vi "key_jiaoyan.vi"(10 "key_client":string, 11 "gonghao":string) -> (0 "jy":bool, 2 "error":errorcluster caption="错误输出")   [LabVIEW 2017, in "Lib_code.lvlib"]
uses:
  Lib_code.lvlib
panel:
  in  "簇":cluster{"key":string, "time":i64}
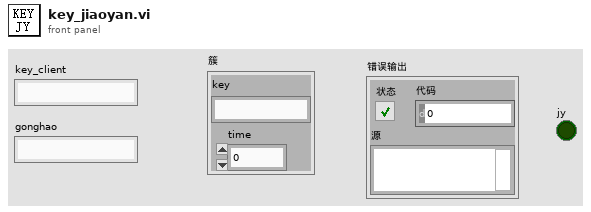
[diagram p1: front panel]
types:
  T1 = enum16{"big-endian, network order", "native, host order", "little-endian"}
  T2 = enum16{"open", "replace", "create", "open or create", "replace or create", "replace or create with confirmation"}
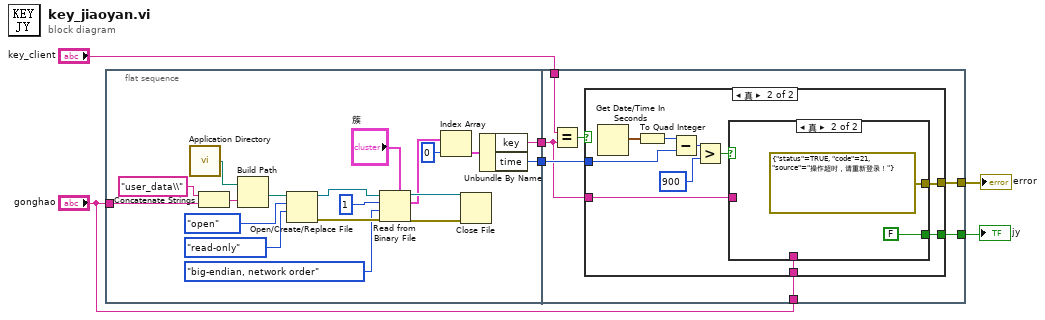
[diagram p0: block diagram]
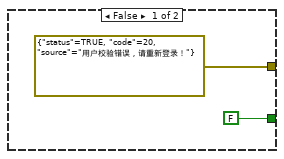
[diagram p2: hidden frame]
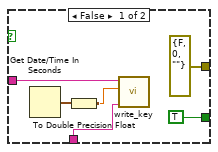
[diagram p3: hidden frame]
diagram:
  n1 = flat-sequence {
    tunnel: "gonghao" -> [w11]
    tunnel: [w10] -> w6
    tunnel: [w9] -> w3
    tunnel: w6 -> [w27]
    tunnel: "key_client" -> [w32]
    tunnel: [w30] -> w4
    tunnel: w3 -> [w29]
    tunnel: [w28] -> w2
    tunnel: "gonghao" -> [w26]
    frame #0 {
      n2 = call <vilib>:"Application Directory.vi"() -> ("Application Directory"=w25:path)
      n3 = Concatenate Strings("user_data\\" ("字符串"), w11) -> (w24:string)
      n4 = Build Path(base path=w25, name or relative path=w24) -> (appended path=w22:path)
      n5 = Open/Create/Replace File(file path (use dialog)=w22, operation (0:open)=T2."open" ("操作(0:open)"), access (0:read/write)=enum16{"read/write", "read-only", "write-only"}."read-only" ("权限(0:read/write)")) -> (refnum out=w17:refnum<file>, error out=w16:errorcluster)  [unwired: 3 in, 1 out]
      n6 = Read from Binary File(5:"簇", 8:w16, 9:T1."big-endian, network order" ("字节顺序(0:big-endian, network order)"), 10:1 ("总数(1)"), 11:w17) -> (0:w19:errorcluster, 2:w14:cluster{"key":string, "time":i64}[], 3:w20:refnum<file>)  [unwired: 1 in, 1 out]
      n7 = Index Array(array=w14, index=0 ("索引")) -> (element=w12:cluster{"key":string, "time":i64})
      n8 = Close File(refnum=w20, error in=w19) -> ()  [unwired: 2 out]
      n9 = Unbundle By Name(w12) -> ("key"=w10:string, "time"=w9:i64)
    }
    frame #1 {
      n10 = Equal?(x=w32, y=w27) -> (x = y?=w31:bool)
      n11 = case shown="真" w31 {
        tunnel: [errorcluster {"status"=TRUE, "code"=20, "source"="用户校验错误，请重新登录！"} ("错误输出") w41] -> w30
        tunnel: w29 -> [_ w44]
        tunnel: [FALSE ("jy") w39] -> w28
        tunnel: w27 -> [_ w38]
        tunnel: w26 -> [_ w37]
        frame False {
        }
        frame True {
          n12 = Get Date/Time In Seconds() -> (seconds since 1Jan1904=w36:timestamp)
          n13 = To Quad Integer(1:w36) -> (0:w35:i64)
          n14 = Subtract(x=w35, y=w44) -> (x-y=w43:i64)
          n15 = Greater?(x=w43, y=i64 900) -> (0:w40:bool)
          n16 = case shown="真" w40 {
            tunnel: [errorcluster {"status"=FALSE, "code"=0, "source"=""} ("错误输出") errorcluster {"status"=TRUE, "code"=21, "source"="操作超时，请重新登录！"} ("错误输出")] -> w41
            tunnel: [TRUE ("jy") FALSE ("jy")] -> w39
            tunnel: w38 -> [w47 _]
            tunnel: w37 -> [w45 _]
            frame False {
              n17 = Get Date/Time In Seconds() -> (seconds since 1Jan1904=w48:timestamp)
              n18 = To Double Precision Float(number=w48) -> (double precision float=w46:dbl)
              n19 = call "write_key.vi"("file_name"=w45, "time"=w46, "key"=w47) -> ()  [unwired: 9 in]
            }
            frame True {
            }
          }
        }
      }
    }
  }
  "error" <- w4
  "jy" <- w2
